vi "test - Basic Function.vi"(8 "error in (no error)":errorcluster, 11 "TestCase in":refnum<class "testcase-Broadcast Registry.lvclass">) -> (0 "error out":errorcluster, 3 "TestCase out":refnum<class "testcase-Broadcast Registry.lvclass">)   [LabVIEW 2017, in "testcase-Broadcast Registry.lvclass"]
uses:
  testcase-Broadcast Registry.lvclass
  f1ab6f25-c30d-499f-96ca-3a55fa643449.vi
  src/user.lib/_NEVSTOP/Communicable State Machine(CSM)/AdvanceAPI/CSM - Revert Arguments-Safe String.vi
  src/user.lib/_NEVSTOP/Communicable State Machine(CSM)/AdvanceAPI/CSM - Make String Arguments Safe.vi
  src/user.lib/_NEVSTOP/Communicable State Machine(CSM)/AdvanceAPI/CSM - Break Down Multiple States String.vi
  src/user.lib/_NEVSTOP/Communicable State Machine(CSM)/AdvanceAPI/CSM - Compact Multiple States.vi
  src/user.lib/_NEVSTOP/Communicable State Machine(CSM)/AdvanceAPI/CSM - Keywords.vi
  src/user.lib/_NEVSTOP/Communicable State Machine(CSM)/_Shared/Trim Single-line Text.vi
  <vilib>/addons/_JKI Toolkits/VI Tester/TestCase.llb/TestCase.lvclass
  src/user.lib/_NEVSTOP/Communicable State Machine(CSM)/Communicable State Machine.lvlib
  C:/Program Files (x86)/National Instruments/LabVIEW 2017/vi.lib/addons/_JKI Toolkits/VI Tester/TestCase.llb/TestCase.lvclass
panel:
  out "Error Occurred":errorcluster
  out "State History":string
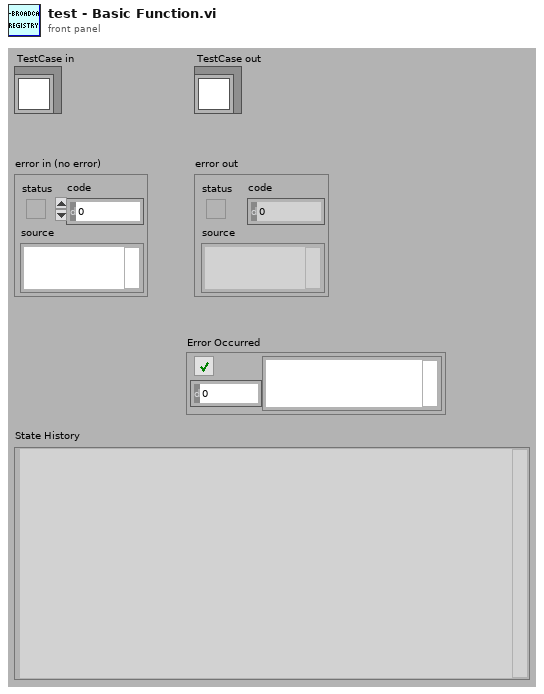
[diagram p1: front panel]
types:
  T1 = enum32{"Invalid", "Standard", "Closed", "Hidden", "Minimized", "Maximized"}
  T2 = enum32{"invalid app kind", "Development System", "Run Time System", "Student Edition", "Embedded LabVIEW", "Evaluation", "Custom"}
  T3 = cluster{"Status":string, "Source CSM":string, "Target CSM":string, "Target API":string}[]
  T4 = typedef "Communicable State Machine.lvlib/_CSM_Response Source Message.ctl" = cluster{"‘State":string, "’Arguments":string, "’Error":errorcluster}
  T5 = cluster{"Current VI Reference":refnum<vi>, "Close Panel on Exit?":bool}
  T6 = cluster{"Core":cluster{"Current VI Reference":refnum<vi>, "Close Panel on Exit?":bool}, "Your Boolean data":bool, "Your string data":string}
  T7 = cluster{"Status":string, "Source CSM":string, "Target CSM":string, "Target API":string}
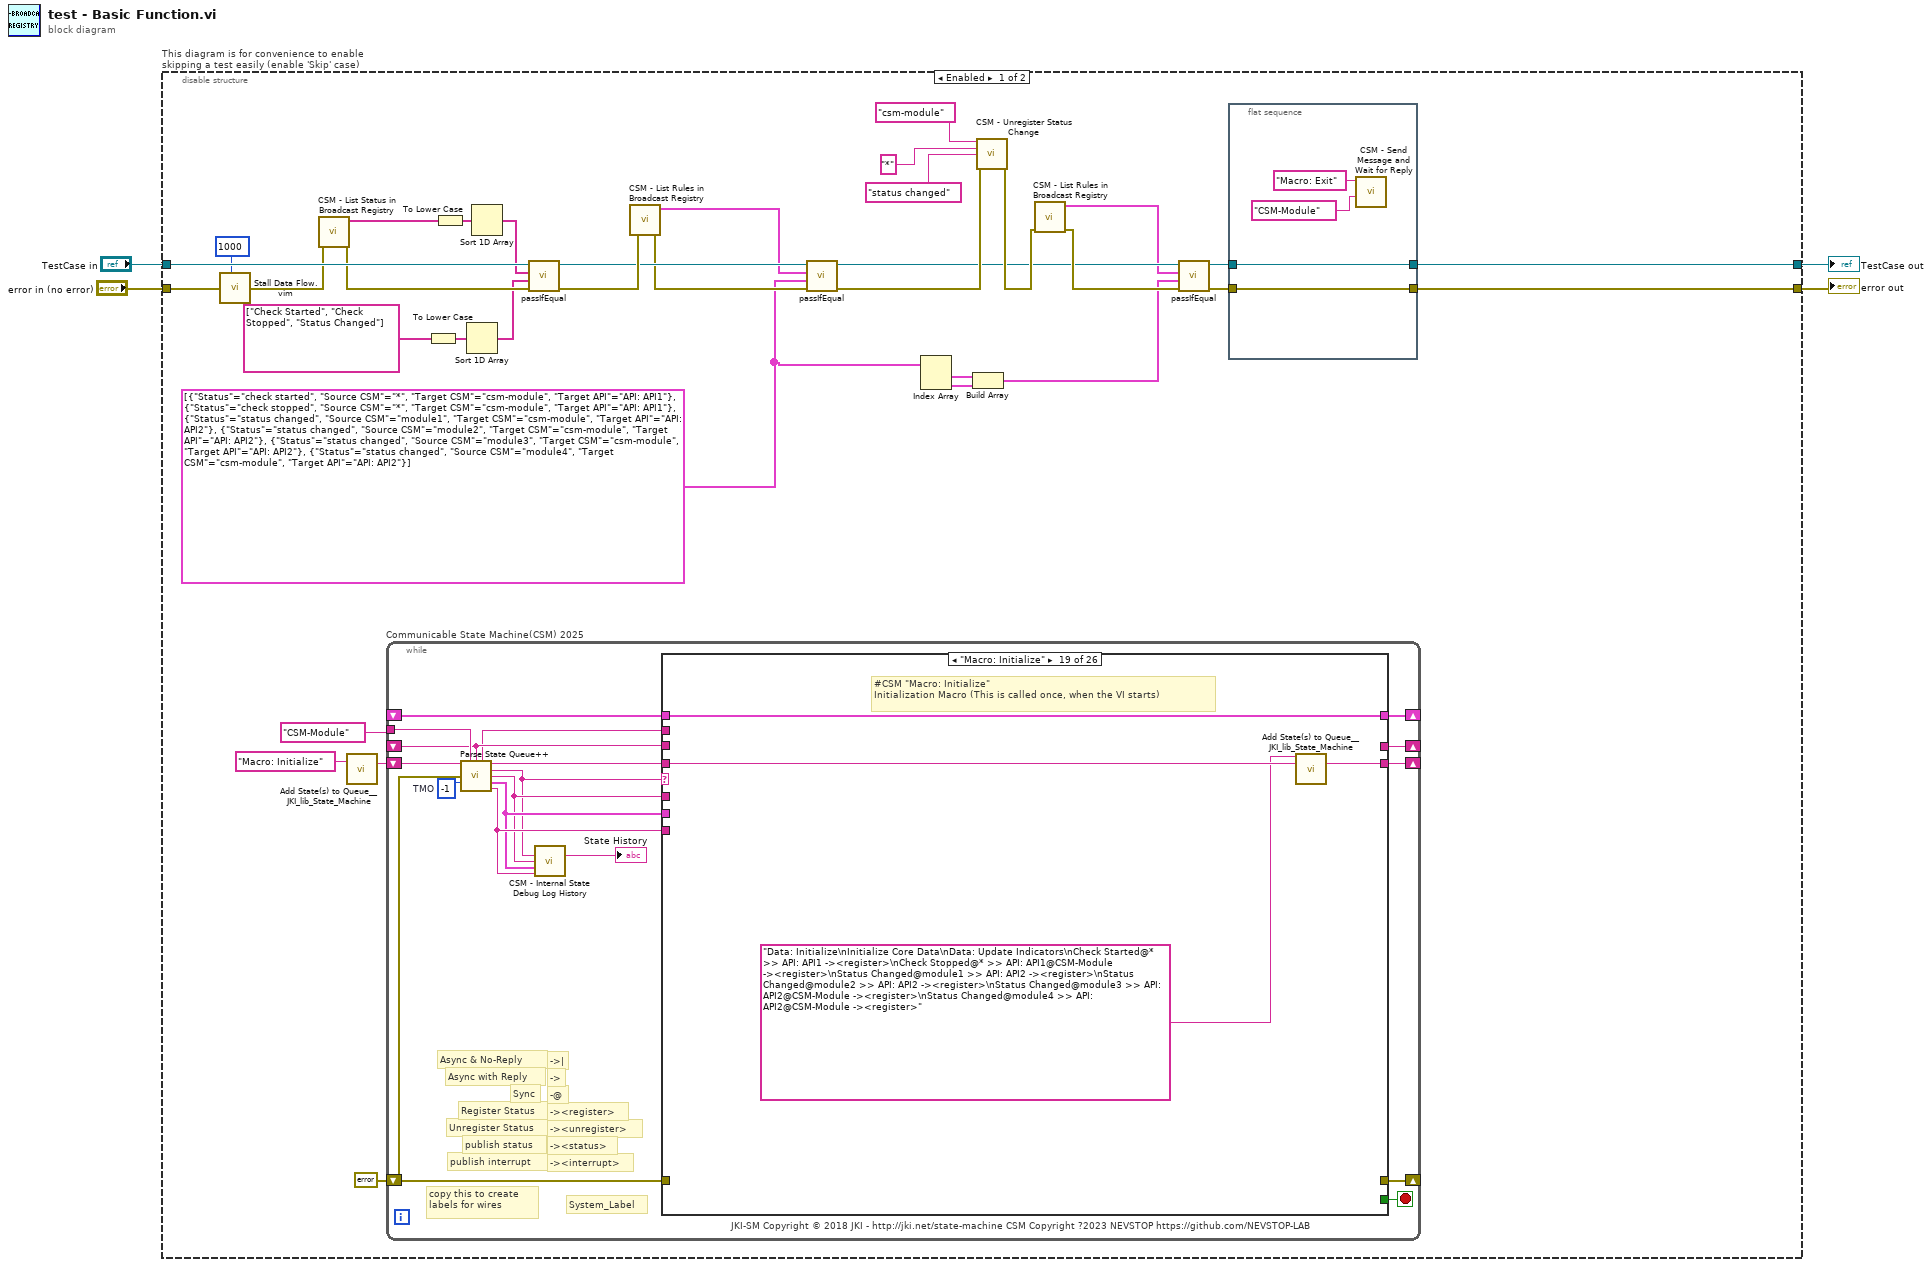
[diagram p0: block diagram]
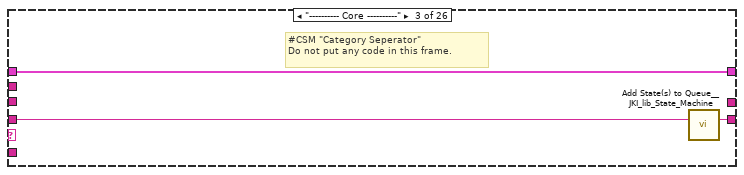
[diagram p4: hidden frame]
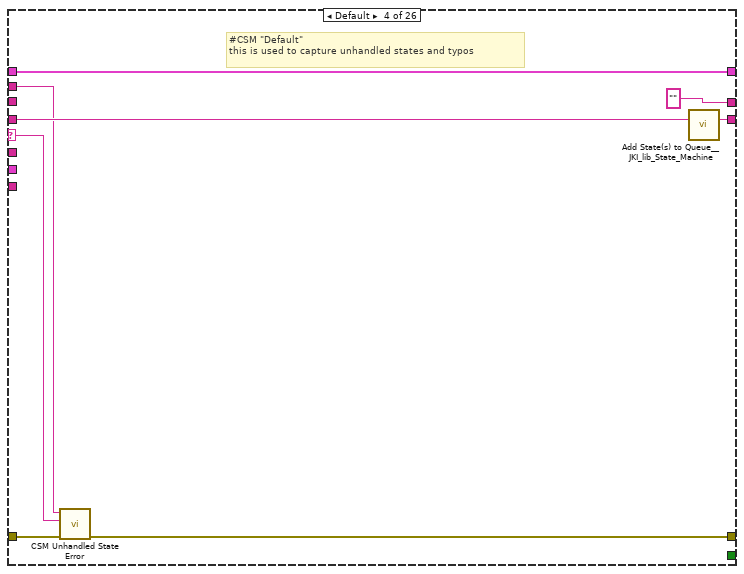
[diagram p5: hidden frame]
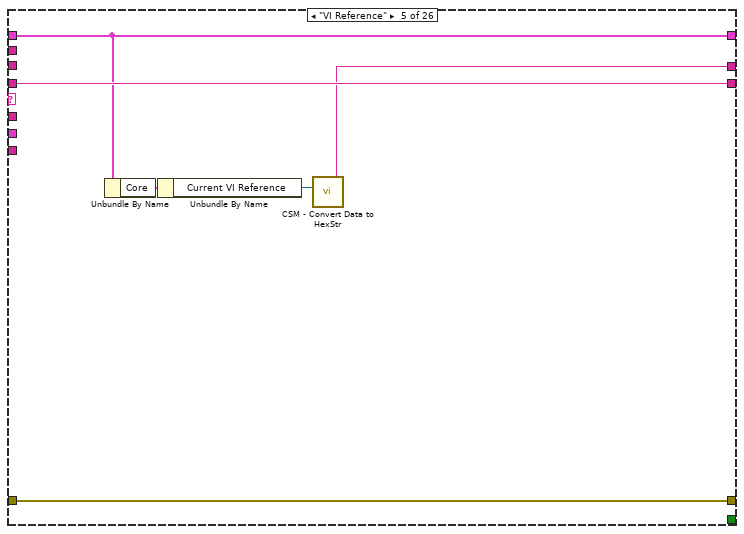
[diagram p6: hidden frame]
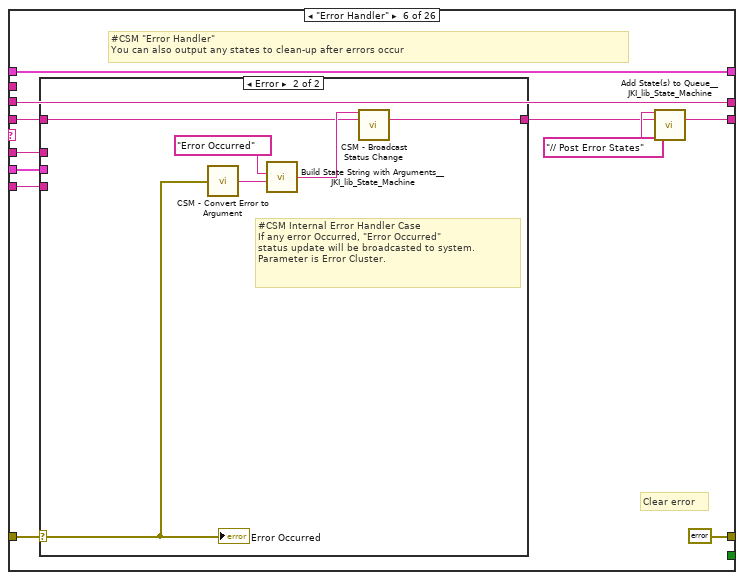
[diagram p7: hidden frame]
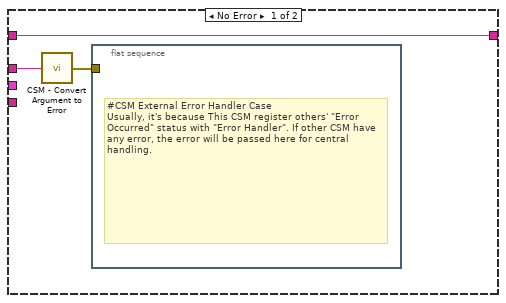
[diagram p8: hidden frame]
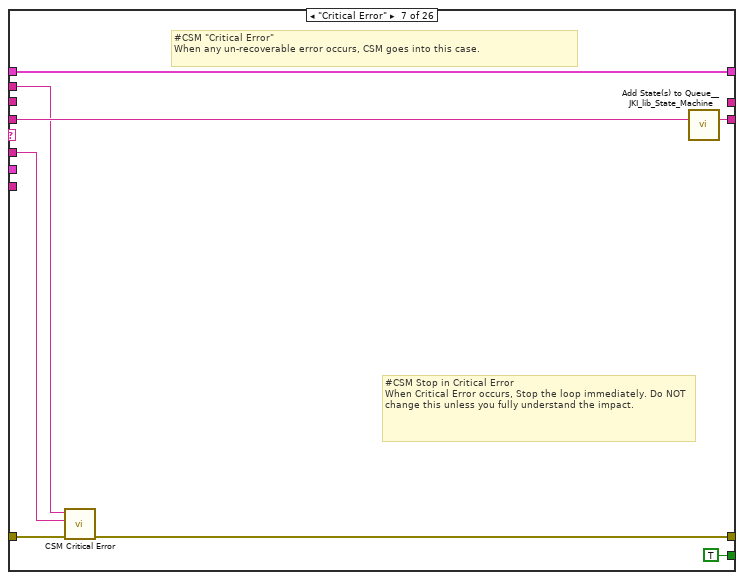
[diagram p9: hidden frame]
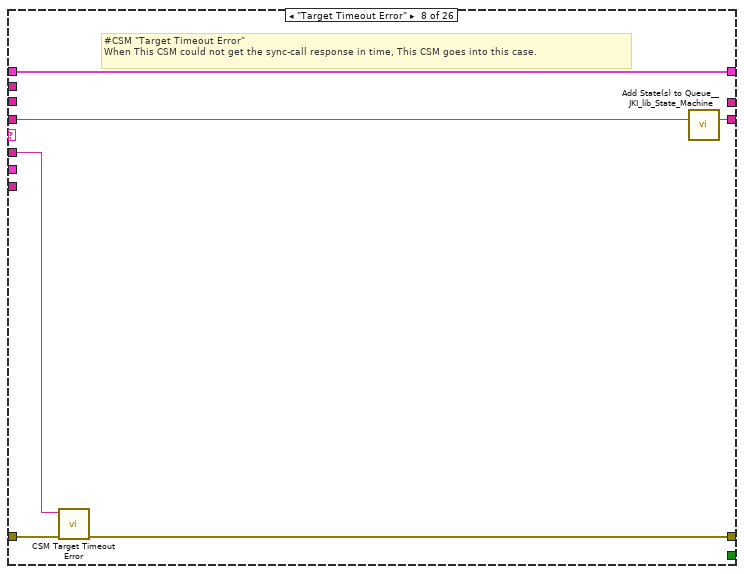
[diagram p10: hidden frame]
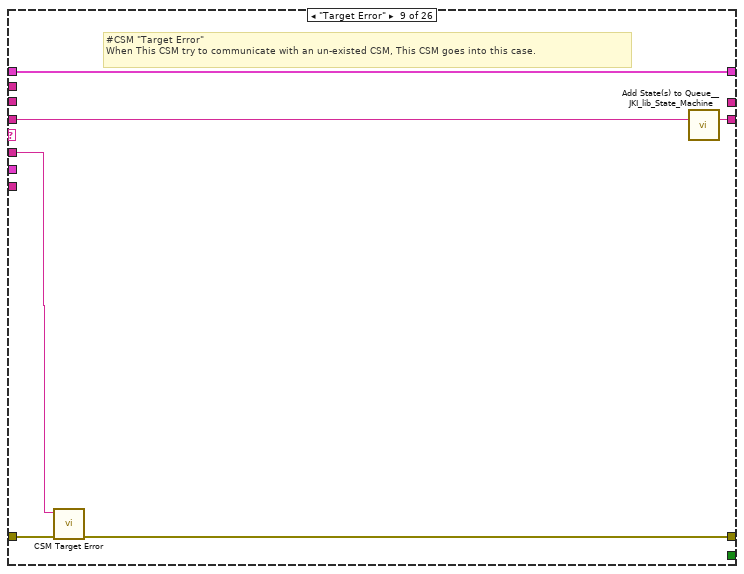
[diagram p11: hidden frame]
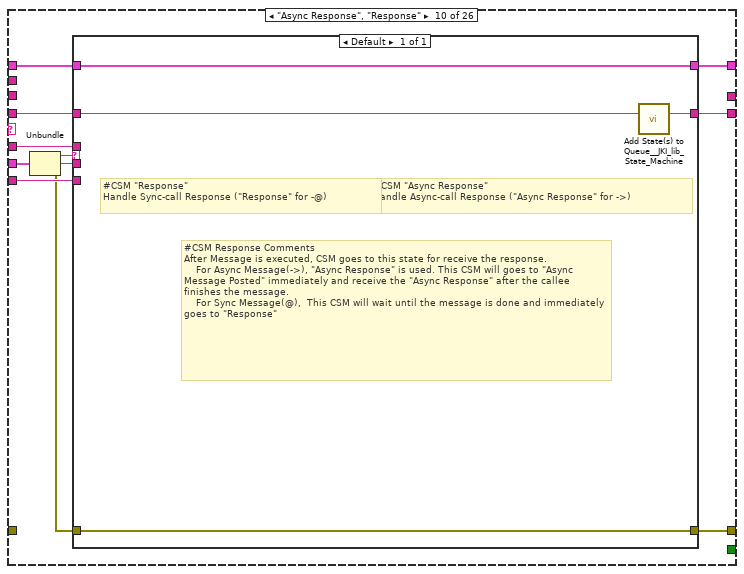
[diagram p12: hidden frame]
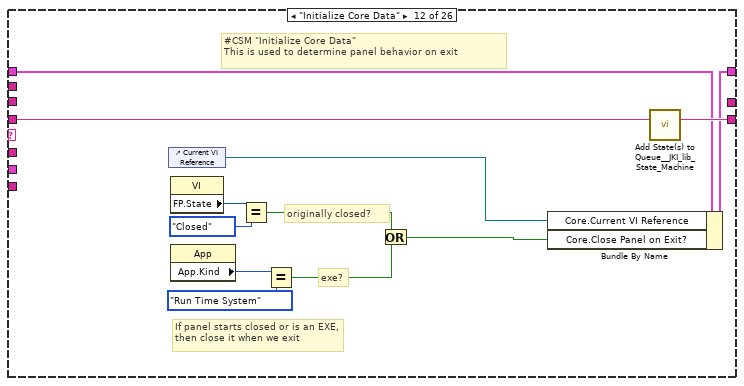
[diagram p14: hidden frame]
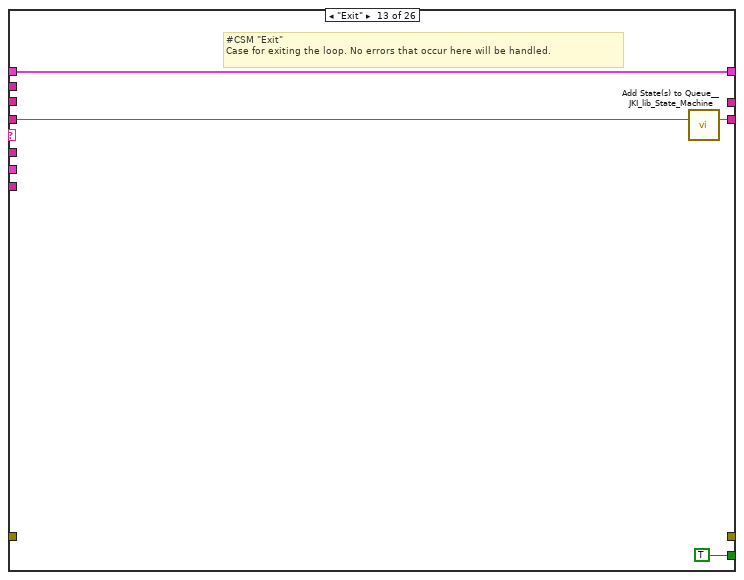
[diagram p15: hidden frame]
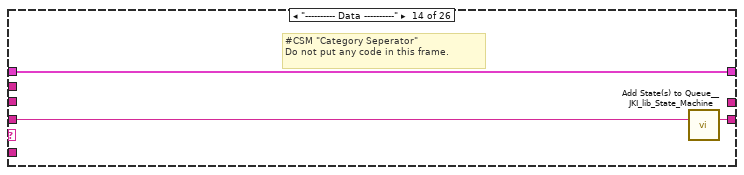
[diagram p16: hidden frame]
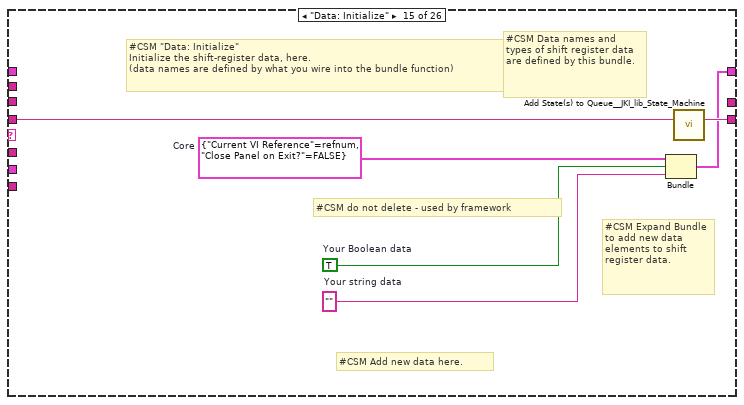
[diagram p17: hidden frame]
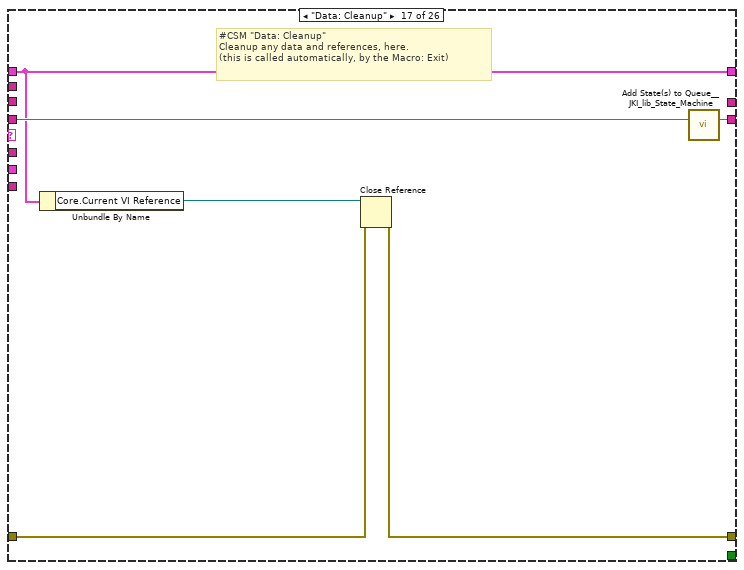
[diagram p19: hidden frame]
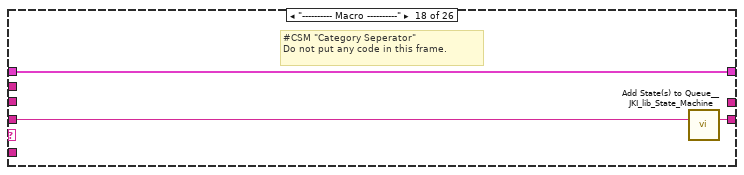
[diagram p20: hidden frame]
diagram:
  n1 = disable-structure "This diagram is for convenience to enable skipping a test easily (enable 'Skip' case)" shown="Enabled" {
    disable-tunnel: "TestCase in" -> [w39 w209]
    disable-tunnel: [w21 w207] -> w1
    disable-tunnel: [w28 w208] -> w3
    disable-tunnel: "error in (no error)" -> [w38 w206]
    frame Enabled {
      w8 = T3 [{"Status"="check started", "Source CSM"="*", "Target CSM"="csm-module", "Target API"="API: API1"}, {"Status"="check stopped", "Source CSM"="*", "Target CSM"="csm-module", "Target API"="API: API1"}, {"Status"="status changed", "Source CSM"="module1", "Target CSM"="csm-module", "Target API"="API: API2"}, {"Status"="status changed", "Source CSM"="module2", "Target CSM"="csm-module", "Target API"="API: API2"}, {"Status"="status changed", "Source CSM"="module3", "Target CSM"="csm-module", "Target API"="API: API2"}, {"Status"="status changed", "Source CSM"="module4", "Target CSM"="csm-module", "Target API"="API: API2"}] ("Entries")
      n2 = call "Stall Data Flow.vim"("value in"=w38, "milliseconds to wait"=u32 1000) -> ("value out"=w33:errorcluster)  [unwired: 1 out]
      n3 = call "CSM - List Status in Broadcast Registry.vi"("error in (no error)"=w33) -> ("error out"=w31:errorcluster, "Status In Registry"=w30:string[])  [unwired: 9 in]
      n4 = call <vilib>:"Add State(s) to Queue__JKI_lib_State_Machine.vi"("State(s) in (\"\")"="Macro: Initialize" ("Init State(\"Macro: Initialize\")")) -> ("States Out"=w37:string)  [unwired: 14 in]
      n5 = while "Communicable State Machine(CSM) 2025" {
        shift-right: [w56] -> _
        shift-left: _ -> [w55]
        shift-right: [w59] -> _
        shift-left: errorcluster {"status"=FALSE, "code"=0, "source"=""} ("error out") -> [w45]
        shift-right: [w58] -> _
        shift-left: w37 -> [w60]
        tunnel: "CSM-Module" ("Name (\"\" to Use UUID)") -> [w52]
        shift-right: [w53] -> _
        shift-left: _ -> [w47]
        stop <- w57 stop-if-true
        w54 = -1  # TMO
        # "-><interrupt>"
        # "-><status>"
        # "-><unregister>"
        # "-><register>"
        # "-@"
        # "->"
        # "->|"
        # "publish interrupt"
        # "publish status"
        # "Unregister Status"
        # "Register Status"
        # "Sync"
        # "Async with Reply"
        # "Async & No-Reply"
        # "JKI-SM Copyright © 2018 JKI - http://jki.net/state-machine CSM Copyright ?2023 NEVSTOP https://github.com/NEVSTOP-LAB"
        # "copy this to create labels for wires"
        # "System_Label"
        n6 = call "Parse State Queue++.vi"("State Queue"=w60, "Name (\"\" to Use UUID)"=w52, "Response Arguments"=w47, "Previous Error"=w45, "Dequeue (1 ms)"=w54) -> ("Name Used"=w46:string, "Remaining States"=w61:string, "Current State"=w48:string, "Arguments"=w49:string, ">> Response Source Message >>"=w50:T4, ">> Source CSM >>"=w51:string)  [unwired: 5 in]
        n7 = call "CSM - Internal State Debug Log History.vi"("State"=w48, "Arguments (\"\")"=w49, ">> Response Source Message >>"=w50, "Source (\"\")"=w51) -> ("Debug Log"=→"State History":string)  [unwired: 11 in]
        n8 = case shown="\"Macro: Initialize\"" w48 {
          selector: w48 -> [_ _ _ w72 _ _ _ _ _ _ _ _ _ _ _ _ _ _ _ _ _ _ _ _ _ _]
          tunnel: w61 -> [w62 w65 w68 w76 w81 w87 w110 w116 w122 w132 w139 w151 w155 w158 w164 w166 w172 w175 w179 w185 w187 w190 w194 w199 w202 w205]
          tunnel: w49 -> [_ _ _ _ _ w86 w106 w113 w119 w126 _ _ _ _ _ _ _ _ _ _ _ _ w192 _ _ _]
          tunnel: w55 -> [w63 w64 w66 w74 w80 w92 w108 w114 w120 w130 w138 w145 w153 w156 _ w165 w167 w173 w177 w183 w186 w189 w193 w197 w200 w203]
          tunnel: [_ _ _ w69 w82 errorcluster {"status"=FALSE, "code"=0, "source"=""} ("error out") w103 w111 w117 w133 _ _ _ _ _ _ w168 _ _ _ _ _ _ _ _ _] -> w59
          tunnel: w45 -> [_ _ _ w70 w82 w90 w104 w112 w118 _ _ _ _ _ _ _ w169 _ _ _ _ _ _ _ _ _]
          tunnel: [w62 w65 w67 w75 w81 w88 w109 w115 w121 w131 w139 w150 w154 w157 w163 w166 w171 w174 w178 w184 w187 w190 w194 w198 w201 w204] -> w58
          tunnel: [_ _ _ _ _ _ TRUE _ _ _ _ _ TRUE _ _ _ _ _ _ _ _ _ _ _ _ _] -> w57
          tunnel: [w63 w64 w66 w74 w80 w92 w108 w114 w120 w129 w138 w149 w153 w156 w162 w165 w167 w173 w177 w183 w186 w189 w193 w197 w200 w203] -> w56
          tunnel: w51 -> [_ _ _ _ _ w85 _ _ _ w127 _ _ _ _ _ _ _ _ _ _ _ _ _ _ _ _]
          tunnel: w50 -> [_ _ _ _ _ w84 _ _ _ w128 _ _ _ _ _ _ _ _ _ _ _ _ _ _ _ _]
          tunnel: [_ _ _ "" w77 w83 _ _ _ _ _ _ _ _ _ _ _ _ _ _ _ "API1 Response" w191 _ _ _] -> w53
          tunnel: w46 -> [_ _ _ w71 _ _ w105 _ _ _ _ _ _ _ _ _ _ _ _ _ _ _ _ _ _ _]
          tunnel: w47 -> [_ _ _ _ _ w83 _ _ _ _ _ _ _ _ _ _ _ _ _ _ _ _ _ _ _ _]
          frame "", "Idle" {
            # "#CSM \"Idle/Event Handler\"\nexecutes when the state queue is empty"
          }
          frame "CSM Documentation" {
            # "#CSM Documentation"
            # "#CSM State Syntax\n\n// Comment line, all text to the right of “//” will be ignored\n// Local Message Example\nDoSth: DoA >> Arguments\n\n// Sync Call Example\nAPI: xxxx >> Arguments -@ TargetModule\n\n// Async Call Example\nAPI: xxxx >> Arguments -> TargetModule\n\n// Async Call without Reply Example\nAPI: xxxx >> Arguments ->| TargetModule\n\n// Broadcast normal status:\nStatus >> StatusArguments  -><status>\n\n// Broadcast Interrupt status:\nInterrupt >> StatusArguments  -><interrupt>\n\n// Register Source Module's status to Handler Module\nStatus@Source Module >> Handler Module@Handler Module -><register>\n\n// Unegister Source Module's status\nStatus@Source Module >> Handler Module -><unregister>"
            # "#CSM README FIRST\n\nCommunicable State Machine(CSM) is a LabVIEW application framework that builds upon JKI State Machine(JKISM). It follows the pattern of JKISM and extends the keywords to describe message communication between modules, including concepts such as Sync-Message, Async-Message, Subscription/Unsubscription of status - essential elements for creating reusable code modules. For more information, please visit the CSM wiki: https://nevstop-lab.github.io/CSM-Wiki/\n\nFor instructions on JKI State Machine, visit: \n    http://jki.net/state-machine/\nFor information about CSM, visit: \n    https://github.com/NEVSTOP-LAB"
            # "#CSM \"Documentation\"\nCase for holding CSM Documenation"
          }
          frame "---------- Core ----------" {
            # "#CSM \"Category Seperator\"\nDo not put any code in this frame."
            n9 = call <vilib>:"Add State(s) to Queue__JKI_lib_State_Machine.vi"("State(s) in (\"\")"=w68) -> ("States Out"=w67:string)  [unwired: 14 in]
          }
          frame Default {
            # "#CSM \"Default\"\nthis is used to capture unhandled states and typos"
            n10 = call "CSM Unhandled State Error.vi"("error in (no error)"=w70, "Current State"=w72, "CSM Name"=w71) -> ("error out"=w69:errorcluster)  [unwired: 8 in]
            n11 = call <vilib>:"Add State(s) to Queue__JKI_lib_State_Machine.vi"("State(s) in (\"\")"=w76) -> ("States Out"=w75:string)  [unwired: 14 in]
          }
          frame "VI Reference" {
            n12 = Unbundle By Name(w80) -> ("Core"=w79:T5)
            n13 = Unbundle By Name(w79) -> ("Current VI Reference"=w78:refnum<vi>)
            n14 = call "CSM - Convert Data to HexStr.vi"("Variant"=w78) -> ("HEX String (0-9,A-F)"=w77:string)  [unwired: 8 in]
          }
          frame "Error Handler" {
            # "#CSM \"Error Handler\"\nYou can also output any states to clean-up after errors occur"
            # "Clear error"
            n15 = case shown="Error" w90 {
              selector: w90 -> [_ w97]
              tunnel: [w96 w99] -> w89
              tunnel: w87 -> [w96 w98]
              tunnel: w86 -> [w95 _]
              tunnel: w85 -> [_ _]
              tunnel: w84 -> [_ _]
              frame No Error {
                n16 = call "CSM - Convert Argument to Error.vi"("Argument"=w95) -> ("Error"=w94:errorcluster)  [unwired: 4 in]
                n17 = flat-sequence {
                  tunnel: w94 -> [_]
                  frame #0 {
                    # "#CSM External Error Handler Case\nUsually, it's because This CSM register others' \"Error Occurred\" status with \"Error Handler\". If other CSM have any error, the error will be passed here for central handling."
                  }
                }
              }
              frame Error {
                # "#CSM Internal Error Handler Case \nIf any error Occurred, \"Error Occurred\" \nstatus update will be broadcasted to system.\nParameter is Error Cluster."
                n18 = call "CSM - Convert Error to Argument.vi"("Error"=w97) -> ("Argument"=w101:string)  [unwired: 4 in]
                n19 = call <vilib>:"Build State String with Arguments__JKI_lib_State_Machine.vi"("Arguments (\"\")"=w101, "State"="Error Occurred" ("Status with Arguments")) -> ("State with Arguments"=w100:string)  [unwired: 4 in]
                n20 = call "CSM - Broadcast Status Change.vi"("Status With Arguments"=w100, "State Queue"=w98) -> ("Remaining States"=w99:string)  [unwired: 13 in]
                "Error Occurred" <- w97
              }
            }
            n21 = call <vilib>:"Add State(s) to Queue__JKI_lib_State_Machine.vi"("State(s) in Front (\"\")"="// Post Error States", "State(s) in (\"\")"=w89) -> ("States Out"=w88:string)  [unwired: 13 in]
          }
          frame "Critical Error" {
            # "#CSM \"Critical Error\"\nWhen any un-recoverable error occurs, CSM goes into this case."
            # "#CSM Stop in Critical Error\nWhen Critical Error occurs, Stop the loop immediately. Do NOT change this unless you fully understand the impact."
            n22 = call "CSM Critical Error.vi"("error in (no error)"=w104, "Arugments (As Reason)"=w106, "CSM Name"=w105) -> ("error out"=w103:errorcluster)  [unwired: 8 in]
            n23 = call <vilib>:"Add State(s) to Queue__JKI_lib_State_Machine.vi"("State(s) in (\"\")"=w110) -> ("States Out"=w109:string)  [unwired: 14 in]
          }
          frame "Target Timeout Error" {
            # "#CSM \"Target Timeout Error\"\nWhen This CSM could not get the sync-call response in time, This CSM goes into this case."
            n24 = call "CSM Target Timeout Error.vi"("error in (no error)"=w112, "Arguments (As CSM Name)"=w113) -> ("error out"=w111:errorcluster)  [unwired: 9 in]
            n25 = call <vilib>:"Add State(s) to Queue__JKI_lib_State_Machine.vi"("State(s) in (\"\")"=w116) -> ("States Out"=w115:string)  [unwired: 14 in]
          }
          frame "Target Error" {
            # "#CSM \"Target Error\"\nWhen This CSM try to communicate with an un-existed CSM, This CSM goes into this case."
            n26 = call "CSM Target Error.vi"("error in (no error)"=w118, "Arguments (As CSM Name)"=w119) -> ("error out"=w117:errorcluster)  [unwired: 9 in]
            n27 = call <vilib>:"Add State(s) to Queue__JKI_lib_State_Machine.vi"("State(s) in (\"\")"=w122) -> ("States Out"=w121:string)  [unwired: 14 in]
          }
          frame "Async Response", "Response" {
            n28 = Unbundle(w128) -> ("‘State"=w125:string, "’Arguments"=w124:string, "’Error"=w123:errorcluster)
            n29 = case shown="Default" w125 {
              tunnel: [w134] -> w131
              tunnel: w132 -> [w135]
              tunnel: [w137] -> w129
              tunnel: w130 -> [w137]
              tunnel: [w136] -> w133
              tunnel: w123 -> [w136]
              tunnel: w127 -> [_]
              tunnel: w126 -> [_]
              tunnel: w124 -> [_]
              frame Default {
                # "#CSM \"Async Response\"\nHandle Async-call Response (\"Async Response\" for ->)"
                # "#CSM \"Response\"\nHandle Sync-call Response (\"Response\" for -@)"
                # "#CSM Response Comments\nAfter Message is executed, CSM goes to this state for receive the response.\n    For Async Message(->), \"Async Response\" is used. This CSM will goes to \"Async Message Posted\" immediately and receive the \"Async Response\" after the callee finishes the message.\n    For Sync Message(@),  This CSM will wait until the message is done and immediately goes to \"Response\""
                n30 = call <vilib>:"Add State(s) to Queue__JKI_lib_State_Machine.vi"("State(s) in (\"\")"=w135) -> ("States Out"=w134:string)  [unwired: 14 in]
              }
            }
          }
          frame "Async Message Posted" {
            # "#CSM \"Async Message Posted\"\nAfter Async Message is posted (-> or ->| ), CSM goes to this state for post-action.\nYou can use Argument - State to tell which Async Message is called."
          }
          frame "Initialize Core Data" {
            # "#CSM \"Initialize Core Data\"\nThis is used to determine panel behavior on exit"
            # "originally closed?"
            # "exe?"
            # "If panel starts closed or is an EXE, then close it when we exit"
            n31 = control-ref of="Current VI Reference"() -> (w143:refnum<vi>)
            n32 = property class="VI"() -> ("FP.State"=w142:T1)  [unwired: 2 in, 2 out]
            n33 = property class="App"() -> ("App.Kind"=w148:T2)  [unwired: 2 in, 2 out]
            n34 = Equal?(x=w142, y=T1."Closed" ("Front Panel Window:State")) -> (x = y?=w140:bool)
            n35 = Equal?(x=w148, y=T2."Run Time System" ("Application:Kind")) -> (x = y?=w146:bool)
            n36 = Or(x=w140, y=w146) -> (x .or. y?=w144:bool)
            n37 = Bundle By Name(cluster=w145, "Core.Current VI Reference"=w143, "Core.Close Panel on Exit?"=w144) -> (w149:T6)
            n38 = call <vilib>:"Add State(s) to Queue__JKI_lib_State_Machine.vi"("State(s) in (\"\")"=w151) -> ("States Out"=w150:string)  [unwired: 14 in]
          }
          frame "Exit" {
            # "#CSM \"Exit\"\nCase for exiting the loop. No errors that occur here will be handled."
            n39 = call <vilib>:"Add State(s) to Queue__JKI_lib_State_Machine.vi"("State(s) in (\"\")"=w155) -> ("States Out"=w154:string)  [unwired: 14 in]
          }
          frame "---------- Data ----------" {
            # "#CSM \"Category Seperator\"\nDo not put any code in this frame."
            n40 = call <vilib>:"Add State(s) to Queue__JKI_lib_State_Machine.vi"("State(s) in (\"\")"=w158) -> ("States Out"=w157:string)  [unwired: 14 in]
          }
          frame "Data: Initialize" {
            w159 = T5 {"Current VI Reference"=refnum, "Close Panel on Exit?"=FALSE}  # Core
            w161 = TRUE  # Your Boolean data
            w160 = ""  # Your string data
            # "#CSM \"Data: Initialize\"\nInitialize the shift-register data, here.\n(data names are defined by what you wire into the bundle function)"
            # "#CSM do not delete - used by framework"
            # "#CSM Expand Bundle to add new data elements to shift register data."
            # "#CSM Add new data here."
            # "#CSM Data names and types of shift register data are defined by this bundle."
            n41 = Bundle("Core"=w159, "Your Boolean data"=w161, "Your string data"=w160) -> (w162:T6)  [unwired: 1 in]
            n42 = call <vilib>:"Add State(s) to Queue__JKI_lib_State_Machine.vi"("State(s) in (\"\")"=w164) -> ("States Out"=w163:string)  [unwired: 14 in]
          }
          frame "Data: Update Indicators" {
          }
          frame "Data: Cleanup" {
            # "#CSM \"Data: Cleanup\"\nCleanup any data and references, here.\n(this is called automatically, by the Macro: Exit)"
            n43 = Unbundle By Name(w167) -> ("Core.Current VI Reference"=w170:refnum<vi>)
            n44 = Close Reference(reference=w170, error in (no error)=w169) -> (error out=w168:errorcluster)
            n45 = call <vilib>:"Add State(s) to Queue__JKI_lib_State_Machine.vi"("State(s) in (\"\")"=w172) -> ("States Out"=w171:string)  [unwired: 14 in]
          }
          frame "---------- Macro ----------" {
            # "#CSM \"Category Seperator\"\nDo not put any code in this frame."
            n46 = call <vilib>:"Add State(s) to Queue__JKI_lib_State_Machine.vi"("State(s) in (\"\")"=w175) -> ("States Out"=w174:string)  [unwired: 14 in]
          }
          frame "Macro: Initialize" {
            # "#CSM \"Macro: Initialize\"\nInitialization Macro (This is called once, when the VI starts)"
            n47 = call <vilib>:"Add State(s) to Queue__JKI_lib_State_Machine.vi"("State(s) in Front (\"\")"="Data: Initialize\nInitialize Core Data\nData: Update Indicators\nCheck Started@* >> API: API1 -><register>\nCheck Stopped@* >> API: API1@CSM-Module -><register>\nStatus Changed@module1 >> API: API2 -><register>\nStatus Changed@module2 >> API: API2 -><register>\nStatus Changed@module3 >> API: API2@CSM-Module -><register>\nStatus Changed@module4 >> API: API2@CSM-Module -><register>", "State(s) in (\"\")"=w179) -> ("States Out"=w178:string)  [unwired: 13 in]
          }
          frame "Macro: Exit" {
            # "#CSM \"Macro: Exit\"\nExit Macro (This is called once, when the VI exits)"
            n48 = call <vilib>:"Add State(s) to Queue__JKI_lib_State_Machine.vi"("State(s) in Front (\"\")"="//Exit Sub-Modules ", "State(s) at Back (\"\")"="Data: Cleanup\nExit") -> ("States Out"=w181:string)  [unwired: 13 in]
            n49 = call <vilib>:"Add State(s) to Queue__JKI_lib_State_Machine.vi"("State(s) in Front (\"\")"=w181, "State(s) in (\"\")"=w185) -> ("States Out"=w184:string)  [unwired: 13 in]
          }
          frame "---------- API ----------" {
            # "#CSM \"Category Seperator\"\nDo not put any code in this frame."
          }
          frame "API: API1" {
            # "#CSM API Example\nCopy/Rename this case for your own API"
            # "#CSM >> Msg/Rep's CSM >>\nIf you need to tell who triggered this state , use this string. If it's this case itself, this string is \"\"."
            # "#CSM >> Arguments >>\nDeal with the parameter if any"
            # "#CSM Response\nConnect this to return the response of your API"
          }
          frame "API: API2" {
            # "#CSM API Example\nCopy/Rename this case for your own API"
            # "unpack Hex String  to Variant\nif complex parameter is needed."
            n50 = call "CSM - Convert HexStr to Data.vi"("HEX String"=w192) -> ()  [unwired: 7 in, 2 out]
            n51 = disable-structure shown="Disabled" {
              disable-tunnel: [w195 "API2 Response"] -> w191
              frame Disabled {
                # "pack variant to hexstr \nif complex response is needed."
                # "complex Response"
                n52 = call "CSM - Convert Data to HexStr.vi"() -> ("HEX String (0-9,A-F)"=w195:string)  [unwired: 9 in]
              }
              frame Enabled {
              }
            }
          }
          frame "---------- Action ----------" {
            # "#CSM \"Category Seperator\"\nDo not put any code in this frame."
            n53 = call <vilib>:"Add State(s) to Queue__JKI_lib_State_Machine.vi"("State(s) in (\"\")"=w199) -> ("States Out"=w198:string)  [unwired: 14 in]
          }
          frame "Action: action1" {
            # "#CSM \"Internal State\"\nThis category is used for holding internal states"
            n54 = call <vilib>:"Add State(s) to Queue__JKI_lib_State_Machine.vi"("State(s) in (\"\")"=w202) -> ("States Out"=w201:string)  [unwired: 14 in]
          }
          frame "Action: action2" {
            # "#CSM \"Internal State\"\nThis category is used for holding internal states"
            n55 = call <vilib>:"Add State(s) to Queue__JKI_lib_State_Machine.vi"("State(s) in (\"\")"=w205) -> ("States Out"=w204:string)  [unwired: 14 in]
          }
        }
      }
      n56 = To Lower Case(string=string[] ["Check Started", "Check Stopped", "Status Changed"] ("Status in Registry")) -> (all lower case string=w25:string[])
      n57 = To Lower Case(string=w30) -> (all lower case string=w24:string[])
      n58 = Sort 1D Array(array=w25) -> (sorted array=w26:string[])
      n59 = Sort 1D Array(array=w24) -> (sorted array=w27:string[])
      n60 = call-dynamic "passIfEqual.vi"("error in (no error)"=w31, "y"=w26, "x"=w27, "TestCase in"=w39) -> ("error out"=w23:errorcluster, "TestCase out"=w22:refnum<class "testcase-Broadcast Registry.lvclass">)  [unwired: 6 in]
      n61 = call "CSM - List Rules in Broadcast Registry.vi"("error in (no error)"=w23) -> ("error out"=w20:errorcluster, "Entries"=w18:T3)  [unwired: 9 in]
      n62 = call-dynamic "passIfEqual.vi"("error in (no error)"=w20, "y"=w8, "x"=w18, "TestCase in"=w22) -> ("error out"=w19:errorcluster, "TestCase out"=w12:refnum<class "testcase-Broadcast Registry.lvclass">)  [unwired: 6 in]
      n63 = Index Array(array=w8) -> (element #1=w7:T7, element #2=w6:T7)  [unwired: 2 in]
      n64 = Build Array(w7, w6) -> (w5:T3)
      n65 = call "CSM - Unregister Status Change.vi"("CSM Name"="csm-module", "Source CSM Name (* as Default)"="*", "Status"="status changed", "Error In"=w19) -> ("error out"=w14:errorcluster)  [unwired: 10 in, 1 out]
      n66 = call "CSM - List Rules in Broadcast Registry.vi"("error in (no error)"=w14) -> ("error out"=w13:errorcluster, "Entries"=w9:T3)  [unwired: 9 in]
      n67 = call-dynamic "passIfEqual.vi"("error in (no error)"=w13, "y"=w5, "x"=w9, "TestCase in"=w12) -> ("error out"=w10:errorcluster, "TestCase out"=w11:refnum<class "testcase-Broadcast Registry.lvclass">)  [unwired: 6 in]
      n68 = flat-sequence {
        tunnel: [w41] -> w28
        tunnel: w10 -> [w41]
        tunnel: [w40] -> w21
        tunnel: w11 -> [w40]
        frame #0 {
          n69 = call "CSM - Send Message and Wait for Reply.vi"("Target Module"="CSM-Module" ("Name (\"\" to Use UUID)"), "State"="Macro: Exit") -> ()  [unwired: 7 in, 3 out]
        }
      }
    }
    frame Disabled {
      # "skip test result while test is under development"
      n70 = call <vilib>:"skip.vi"("error in (no error)"=w206, "TestCase in"=w209) -> ("error out"=w208:errorcluster, "TestCase out"=w207:refnum<class "testcase-Broadcast Registry.lvclass">)  [unwired: 8 in]
    }
  }
  "error out" <- w3
  "TestCase out" <- w1
